vi "Get Temperature Coefficient Frequencies.vi"(0 "VISA resource name":refnum<visa-resource-name>="USB0::0x2226::0x000F::00000000::INSTR", 11 "error in (no error)":errorcluster) -> (4 "VISA resource name out":refnum<visa-resource-name>, 8 "Temp Coefficient Frequencies":dbl[](array[numeric])=[100000.0, 22599750.0, 45099500.0, 67599250.0, 90099000.0, 112598750.0, 135098500.0, 157598250.0, 180098000.0, 202597750.0, 225097500.0, 247597250.0, 270097000.0, 292596750.0, 315096500.0, 337596250.0, 360096000.0, 382595750.0, 405095500.0, 427595250.0, 450095000.0, 472594750.0, 495094500.0, 517594250.0, 540094000.0, 562593750.0, 585093500.0, 607593250.0, 630093000.0, 652592750.0, 675092500.0, 697592250.0, 720092000.0, 742591750.0, 765091500.0, 787591250.0, 810091000.0, 832590750.0, 855090500.0, 877590250.0, 900090000.0, 922589750.0, 945089500.0, 967589250.0, 990089000.0, 1012588750.0, 1035088500.0, 1057588250.0, 1080088000.0, 1102587750.0, 1125087500.0, 1147587250.0, 1170087000.0, 1192586750.0, 1215086500.0, 1237586250.0, 1260086000.0, 1282585750.0, 1305085500.0, 1327585250.0, 1350085000.0, 1372584750.0, 1395084500.0, 1417584250.0, 1440084000.0, 1462583750.0, 1485083500.0, 1507583250.0, 1530083000.0, 1552582750.0, 1575082500.0, 1597582250.0, 1620082000.0, 1642581750.0, 1665081500.0, 1687581250.0, 1710081000.0, 1732580750.0, 1755080500.0, 1777580250.0, 1800080000.0, 1822579750.0, 1845079500.0, 1867579250.0, 1890079000.0, 1912578750.0, 1935078500.0, 1957578250.0, 1980078000.0, 2002577750.0, 2025077500.0, 2047577250.0, 2070077000.0, 2092576750.0, 2115076500.0, 2137576250.0, 2160076000.0, 2182575750.0, 2205075500.0, 2227575250.0, 2250075000.0, 2272574750.0, 2295074500.0, 2317574250.0, 2340074000.0, 2362573750.0, 2385073500.0, 2407573250.0, 2430073000.0, 2452572750.0, 2475072500.0, 2497572250.0, 2520072000.0, 2542571750.0, 2565071500.0, 2587571250.0, 2610071000.0, 2632570750.0, 2655070500.0, 2677570250.0, 2700070000.0, 2722569750.0, 2745069500.0, 2767569250.0, 2790069000.0, 2812568750.0, 2835068500.0, 2857568250.0, 2880068000.0, 2902567750.0, 2925067500.0, 2947567250.0, 2970067000.0, 2992566750.0, 3015066500.0, 3037566250.0, 3060066000.0, 3082565750.0, 3105065500.0, 3127565250.0, 3150065000.0, 3172564750.0, 3195064500.0, 3217564250.0, 3240064000.0, 3262563750.0, 3285063500.0, 3307563250.0, 3330063000.0, 3352562750.0, 3375062500.0, 3397562250.0, 3420062000.0, 3442561750.0, 3465061500.0, 3487561250.0, 3510061000.0, 3532560750.0, 3555060500.0, 3577560250.0, 3600060000.0, 3622559750.0, 3645059500.0, 3667559250.0, 3690059000.0, 3712558750.0, 3735058500.0, 3757558250.0, 3780058000.0, 3802557750.0, 3825057500.0, 3847557250.0, 3870057000.0, 3892556750.0, 3915056500.0, 3937556250.0, 3960056000.0, 3982555750.0, 4005055500.0, 4027555250.0, 4050055000.0, 4072554750.0, 4095054500.0, 4117554250.0, 4140054000.0, 4162553750.0, 4185053500.0, 4207553250.0, 4230053000.0, 4252552750.0, 4275052500.0, 4297552250.0, 4320052000.0, 4342551750.0, 4365051500.0, 4387551250.0, 4410051000.0, 4432550750.0, 4455050500.0, 4477550250.0, 4500050000.0, 4522549750.0, 4545049500.0, 4567549250.0, 4590049000.0, 4612548750.0, 4635048500.0, 4657548250.0, 4680048000.0, 4702547750.0, 4725047500.0, 4747547250.0, 4770047000.0, 4792546750.0, 4815046500.0, 4837546250.0, 4860046000.0, 4882545750.0, 4905045500.0, 4927545250.0, 4950045000.0, 4972544750.0, 4995044500.0, 5017544250.0, 5040044000.0, 5062543750.0, 5085043500.0, 5107543250.0, 5130043000.0, 5152542750.0, 5175042500.0, 5197542250.0, 5220042000.0, 5242541750.0, 5265041500.0, 5287541250.0, 5310041000.0, 5332540750.0, 5355040500.0, 5377540250.0, 5400040000.0, 5422539750.0, 5445039500.0, 5467539250.0, 5490039000.0, 5512538750.0, 5535038500.0, 5557538250.0, 5580038000.0, 5602537750.0, 5625037500.0, 5647537250.0, 5670037000.0, 5692536750.0, 5715036500.0, 5737536250.0, 5760036000.0, 5782535750.0, 5805035500.0, 5827535250.0, 5850035000.0, 5872534750.0, 5895034500.0, 5917534250.0, 5940034000.0, 5962533750.0, 5985033500.0, 6007533250.0, 6030033000.0, 6052532750.0, 6075032500.0, 6097532250.0, 6120032000.0, 6142531750.0, 6165031500.0, 6187531250.0, 6210031000.0, 6232530750.0, 6255030500.0, 6277530250.0, 6300030000.0, 6322529750.0, 6345029500.0, 6367529250.0, 6390029000.0, 6412528750.0, 6435028500.0, 6457528250.0, 6480028000.0, 6502527750.0, 6525027500.0, 6547527250.0, 6570027000.0, 6592526750.0, 6615026500.0, 6637526250.0, 6660026000.0, 6682525750.0, 6705025500.0, 6727525250.0, 6750025000.0, 6772524750.0, 6795024500.0, 6817524250.0, 6840024000.0, 6862523750.0, 6885023500.0, 6907523250.0, 6930023000.0, 6952522750.0, 6975022500.0, 6997522250.0, 7020022000.0, 7042521750.0, 7065021500.0, 7087521250.0, 7110021000.0, 7132520750.0, 7155020500.0, 7177520250.0, 7200020000.0, 7222519750.0, 7245019500.0, 7267519250.0, 7290019000.0, 7312518750.0, 7335018500.0, 7357518250.0, 7380018000.0, 7402517750.0, 7425017500.0, 7447517250.0, 7470017000.0, 7492516750.0, 7515016500.0, 7537516250.0, 7560016000.0, 7582515750.0, 7605015500.0, 7627515250.0, 7650015000.0, 7672514750.0, 7695014500.0, 7717514250.0, 7740014000.0, 7762513750.0, 7785013500.0, 7807513250.0, 7830013000.0, 7852512750.0, 7875012500.0, 7897512250.0, 7920012000.0, 7942511750.0, 7965011500.0, 7987511250.0, 8010011000.0, 8032510750.0, 8055010500.0, 8077510250.0, 8100010000.0, 8122509750.0, 8145009500.0, 8167509250.0, 8190009000.0, 8212508750.0, 8235008500.0, 8257508250.0, 8280008000.0, 8302507750.0, 8325007500.0, 8347507250.0, 8370007000.0, 8392506750.0, 8415006500.0, 8437506250.0, 8460006000.0, 8482505750.0, 8505005500.0, 8527505250.0, 8550005000.0, 8572504750.0, 8595004500.0, 8617504250.0, 8640004000.0, 8662503750.0, 8685003500.0, 8707503250.0, 8730003000.0, 8752502750.0, 8775002500.0, 8797502250.0, 8820002000.0, 8842501750.0, 8865001500.0, 8887501250.0, 8910001000.0, 8932500750.0, 8955000500.0, 8977500250.0, 9000000000.0], 15 "error out":errorcluster)   [LabVIEW 2023, in "ACM Visa Driver.lvlib"]
uses:
  ACM Visa Driver.lvlib
  <vilib>/Analysis/1siggen.llb/Ramp Pattern by Samples.vi
  <vilib>/Analysis/NI_AALBase.lvlib
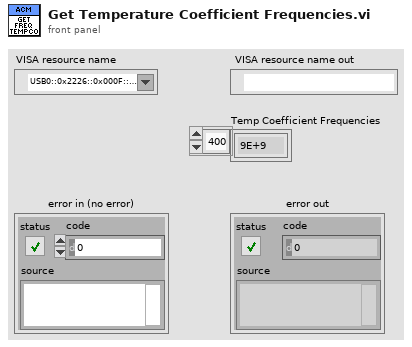
[diagram p1: front panel]
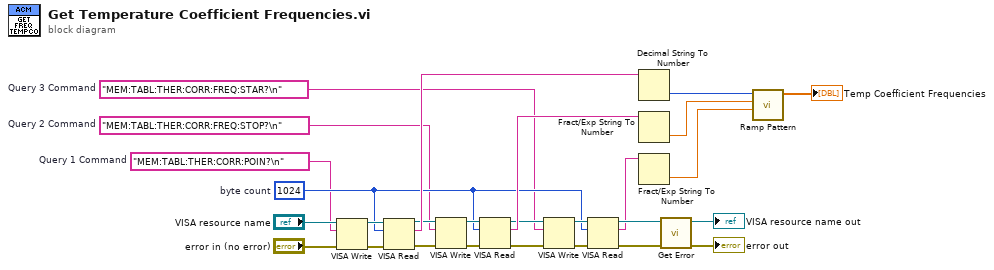
[diagram p0: block diagram]
diagram:
  w1 = "MEM:TABL:THER:CORR:FREQ:STAR?\n"  # Query 3 Command
  w2 = "MEM:TABL:THER:CORR:FREQ:STOP?\n"  # Query 2 Command
  w3 = "MEM:TABL:THER:CORR:POIN?\n"  # Query 1 Command
  w9 = u32 1024  # byte count
  n1 = VISA Write(VISA resource name="VISA resource name", write buffer=w3, error in (no error)="error in (no error)") -> (VISA resource name out=w24:refnum<visa-resource-name>, error out=w25:errorcluster)  [unwired: 1 out]
  n2 = VISA Read(VISA resource name=w24, byte count=w9, error in (no error)=w25) -> (VISA resource name out=w17:refnum<visa-resource-name>, read buffer=w21:string, error out=w18:errorcluster)  [unwired: 1 out]
  n3 = VISA Write(VISA resource name=w17, write buffer=w2, error in (no error)=w18) -> (VISA resource name out=w20:refnum<visa-resource-name>, error out=w19:errorcluster)  [unwired: 1 out]
  n4 = VISA Read(VISA resource name=w20, byte count=w9, error in (no error)=w19) -> (VISA resource name out=w13:refnum<visa-resource-name>, read buffer=w16:string, error out=w14:errorcluster)  [unwired: 1 out]
  n5 = VISA Write(VISA resource name=w13, write buffer=w1, error in (no error)=w14) -> (VISA resource name out=w12:refnum<visa-resource-name>, error out=w15:errorcluster)  [unwired: 1 out]
  n6 = VISA Read(VISA resource name=w12, byte count=w9, error in (no error)=w15) -> (VISA resource name out=w11:refnum<visa-resource-name>, read buffer=w8:string, error out=w10:errorcluster)  [unwired: 1 out]
  n7 = Decimal String To Number(string=w21) -> (number=w7:i32)  [unwired: 2 in, 1 out]
  n8 = Fract/Exp String To Number(string=w16) -> (number=w6:dbl)  [unwired: 3 in, 1 out]
  n9 = Fract/Exp String To Number(string=w8) -> (number=w5:dbl)  [unwired: 3 in, 1 out]
  n10 = call "Get Error.vi"("VISA resource name"=w11, "error in (no error)"=w10) -> ("VISA resource name out"=→"VISA resource name out":refnum<visa-resource-name>, "error out"=→"error out":errorcluster)  [unwired: 12 in]
  n11 = call-poly <vilib>:"Ramp Pattern.vi"("start"=w5, "end"=w6, "samples"=w7) -> ("Ramp Pattern"=→"Temp Coefficient Frequencies":dbl[])  [unwired: 7 in, 1 out]
